vi "distance_from_origin.vi"(10 "y":ext, 11 "x":ext) -> (3 "原点からの距離":ext=20.418127706656477884 format="%#_10g")   [LabVIEW 2020]
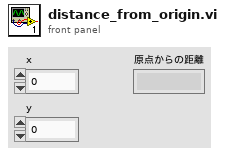
[diagram p1: front panel]
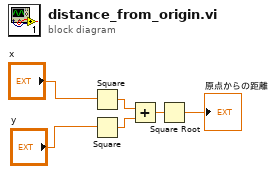
[diagram p0: block diagram]
diagram:
  n1 = Square(x="x") -> (x^2=w4:ext)
  n2 = Square(x="y") -> (x^2=w5:ext)
  n3 = Add(x=w4, y=w5) -> (x+y=w3:ext)
  n4 = Square Root(x=w3) -> (sqrt(x)=→"原点からの距離":ext)
